vi "Test HTTPS.vi"() -> ()   [LabVIEW 2020]
uses:
  lv-http-server/HTTP Server/Trace Log.ctl
  lv-http-server/HTTP Server/Trace Item.ctl
  lv-http-server/HTTP Server/Processing Step.ctl
  lv-http-util/HTTP Utils/Method.ctl
  lv-http-server/HTTP Server/HTTPS Options.ctl
  Test HTTPS Controller/Test HTTPS Controller.lvclass
  C:/dev/lv20CE/relink/lv-http-server/HTTP Server/Handler/Handler.lvclass
  lv-http-server/HTTP Server/Server/Add Connection Handler.vi
  lv-http-server/HTTP Server/Server/Add Request Handler.vi
  lv-http-server/HTTP Server/Server/Add Route Handler.vi
  lv-http-server/HTTP Server/Server/Add Controller Handler.vi
  lv-http-server/HTTP Server/Server/Add Controller.vi
  lv-http-server/HTTP Server/Server/Add Response Handler.vi
  lv-http-server/HTTP Server/Server/Add Complete Handler.vi
  lv-http-server/HTTP Server/Server/Add Exception Handler.vi
  lv-http-server/HTTP Server/Connection Handler/Connection Handler.lvclass
  lv-http-server/HTTP Server/Request Handler/Request Handler.lvclass
  lv-http-server/HTTP Server/Route Handler/Route Handler.lvclass
  lv-http-server/HTTP Server/Controller Handler/Controller Handler.lvclass
  lv-http-server/HTTP Server/Controller/Controller.lvclass
  lv-http-server/HTTP Server/Response Handler/Response Handler.lvclass
  lv-http-server/HTTP Server/Complete Handler/Complete Handler.lvclass
  lv-http-server/HTTP Server/Exception Handler/Exception Handler.lvclass
  lv-http-server/HTTP Server/Server/Server.lvclass
  lv-http-server/HTTP Server/Handler/Handler.lvclass
  lv-http-server/HTTP Server/RequestTraceLog/RequestTraceLog.lvclass
  lv-http-server/HTTP Server/HTTP Server.lvlib
  lv-http-util/HTTP Utils/HTTP Utils.lvlib
panel:
  in  "Public Chain":path=path "C:/dev/lv20CE/relink/lv-http-server-examples/Examples/HTTPS/cert.pem"
  out "error out":errorcluster
  in  "Debug":bool=TRUE
  in  "Refresh Traces":bool
  out "Traces":T1[](array[typedef])=[{"Items"=[{"Duration"=0.00019280000014987309, "Step"=enum."Connection", "Class"="", "Info"="Start Request Parsing", "Status"=FALSE, "Code"=0, "Time"=3234.2736639}, {"Duration"=104.21120999999994, "Step"=enum."Connection", "Class"="", "Info"="Request Initialized", "Status"=TRUE, "Code"=66, "Time"=3338.4848739}, {"Duration"=0.0007422999997288571, "Step"=enum."Connection", "Class"="HTTP Utils.lvlib:Response.lvclass", "Info"="Completed", "Status"=TRUE, "Code"=66, "Time"=3338.4856161999996}], "Client"="tcp://DAB-2020SP1x86.ni.corp.natinst.com:52788", "Target"="", "Response Type"="", "Processing"=0.0007728000000497559, "Status"=200, "Method"=enum."GET", "Content Type"="", "Request Headers"=[], "Parsing"=3338.4848739, "Waiting"=-3234.2736639, "Identity"="", "Loaded"=FALSE, "Created"=FALSE, "Destroyed"=FALSE, "Response Headers"=[], "Created"=0.0, "Expires"=0.0, "Roles"=[], "Sending"=0.0}, {"Items"=[{"Duration"=0.006463199999870994, "Step"=enum."Connection", "Class"="", "Info"="Start Request Parsing", "Status"=FALSE, "Code"=0, "Time"=3459.3199179}, {"Duration"=0.008297200000015437, "Step"=enum."Connection", "Class"="", "Info"="Request Initialized", "Status"=TRUE, "Code"=66, "Time"=3459.3282151}, {"Duration"=0.0001554000000396627, "Step"=enum."Connection", "Class"="HTTP Utils.lvlib:Response.lvclass", "Info"="Completed", "Status"=TRUE, "Code"=66, "Time"=3459.3283705}], "Client"="tcp://DAB-2020SP1x86.ni.corp.natinst.com:52995", "Target"="", "Response Type"="", "Processing"=0.00019930000007661874, "Status"=200, "Method"=enum."GET", "Content Type"="", "Request Headers"=[], "Parsing"=3459.3282151, "Waiting"=-3459.3199179, "Identity"="", "Loaded"=FALSE, "Created"=FALSE, "Destroyed"=FALSE, "Response Headers"=[], "Created"=0.0, "Expires"=0.0, "Roles"=[], "Sending"=0.0}] {"Sending" format="%_6f"; "Expires" format="%<%X %x>T"; "Created" format="%<%X %x>T"; "Waiting" format="%_6f"; "Parsing" format="%_6f"; "Processing" format="%_6f"; "Items"."Time" format="%.6f"; "Items"."Duration" format="%.6f"}
  in  "Private Key":path=path "C:/dev/lv20CE/relink/lv-http-server-examples/Examples/HTTPS/key.pem"
  in  "HTTPS Port":u16=443
  in  "HTTP Port":u16=80
  in  "Always Secure?":bool=TRUE
  # "Request"
  # "Response"
  # "Session"
  # "Auth"
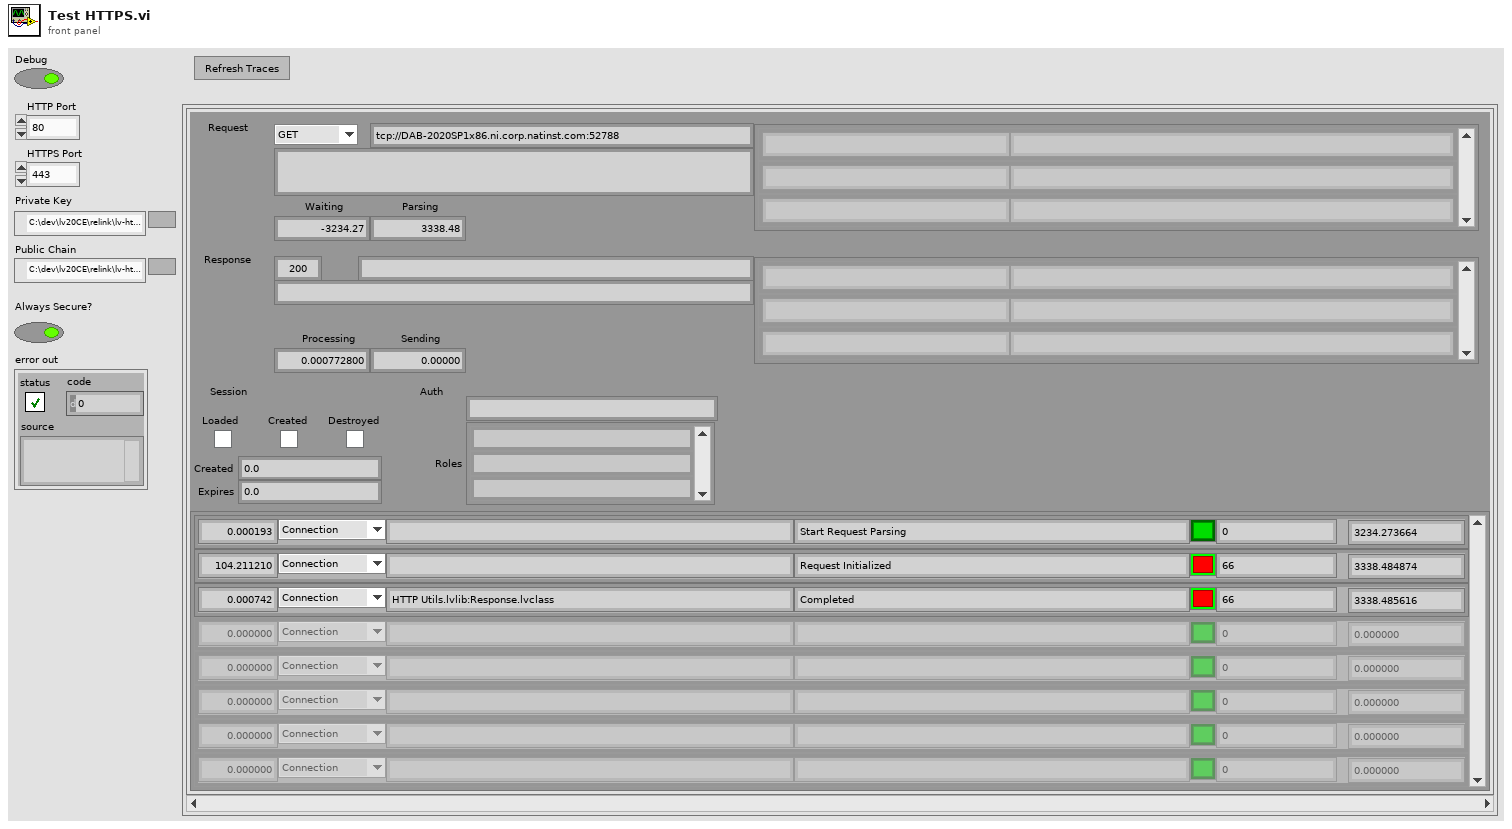
[diagram p1: front panel]
types:
  T1 = typedef "HTTP Server.lvlib/Trace Log.ctl" = cluster{"Items":T2[], "Client":string, "Target":string, "Response Type":string, "Processing":dbl, "Status":u16, "Method":T4, "Content Type":string, "Request Headers":cluster{"Name":string, "Value":string}[], "Parsing":dbl, "Waiting":dbl, "Identity":string, "Loaded":bool, "Created":bool, "Destroyed":bool, "Response Headers":cluster{"Name":string, "Value":string}[], "Created":dbl, "Expires":dbl, "Roles":string[], "Sending":dbl}
  T2 = typedef "HTTP Server.lvlib/Trace Item.ctl" = cluster{"Duration":dbl, "Step":T3, "Class":string, "Info":string, "Status":bool, "Code":i32, "Time":dbl}
  T3 = typedef "HTTP Server.lvlib/Processing Step.ctl" = enum16{"Connection", "Request", "Routing", "Controller Init", "Controller", "Response", "Complete", "Exception"}
  T4 = typedef "HTTP Utils.lvlib/Method.ctl" = enum16{"GET", "HEAD", "POST", "PUT", "DELETE", "CONNECT", "OPTIONS", "TRACE", "PATCH"}
  T5 = typedef "HTTP Server.lvlib/HTTPS Options.ctl" = cluster{"HTTPS Enabled":bool, "Private Key":path, "Private Key Format":enum32{"PKCS#8 (PEM)", "PKCS#8 (DER)"}, "Public Cert":path, "Public Cert Format":enum32{"X.509 (PEM)"}, "Always Secure?":bool, "HTTPS Port (443)":u16}
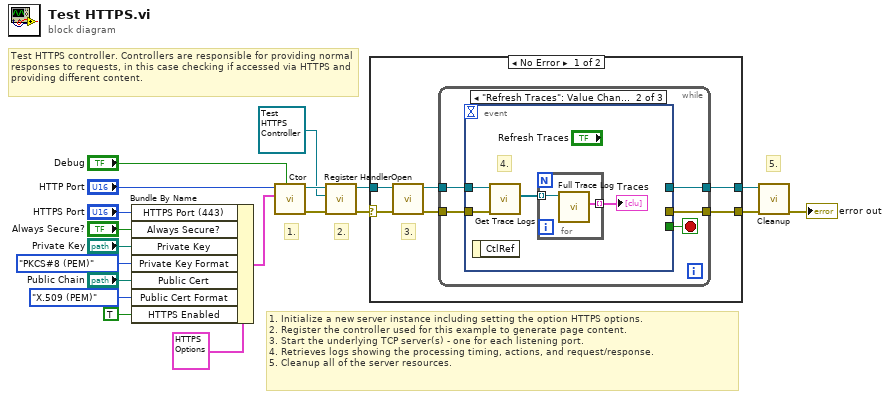
[diagram p0: block diagram]
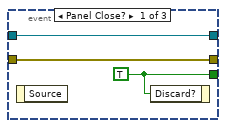
[diagram p2: hidden frame]
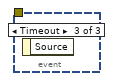
[diagram p3: hidden frame]
diagram:
  # "1. Initialize a new server instance including setting the option HTTPS options.\n2. Register the controller used for this example to generate page content.\n3. Start the underlying TCP server(s) - one for each listening port.\n4. Retrieves logs showing the processing timing, actions, and request/response.\n5. Cleanup all of the server resources."
  # "5."
  # "2."
  # "1."
  # "Test HTTPS controller. Controllers are responsible for providing normal responses to requests, in this case checking if accessed via HTTPS and providing different content."
  n1 = Bundle By Name(cluster=T5 {"HTTPS Enabled"=FALSE, "Private Key"=path "", "Private Key Format"=enum."PKCS#8 (PEM)", "Public Cert"=path "", "Public Cert Format"=enum."X.509 (PEM)", "Always Secure?"=TRUE, "HTTPS Port (443)"=433} ("HTTPS Options"), "HTTPS Port (443)"="HTTPS Port", "Always Secure?"="Always Secure?", "Private Key"="Private Key", "Private Key Format"=enum32{"PKCS#8 (PEM)", "PKCS#8 (DER)"}."PKCS#8 (PEM)", "Public Cert"="Public Chain", "Public Cert Format"=enum32{"X.509 (PEM)"}."X.509 (PEM)" ("Public Chain Format"), "HTTPS Enabled"=TRUE) -> (w4:T5)
  n2 = call "Ctor.vi"("Debug (F)"="Debug", "HTTPS Options (Disabled)"=w4, "HTTP Port (80)"="HTTP Port") -> ("error out"=w18:errorcluster, "Server out"=w19:refnum<class "Server.lvclass">)  [unwired: 7 in]
  n3 = call "Register Handler.vi"("error in (no error)"=w18, "Handler"=refnum<class "Test HTTPS Controller.lvclass"> refnum ("Test HTTPS Controller.lvclass"), "Server in"=w19) -> ("error out"=w1:errorcluster, "Server out"=w2:refnum<class "Server.lvclass">)  [unwired: 7 in]
  n4 = case shown="No Error" w1 {
    selector: w1 -> [w25 w41]
    tunnel: [w22 w40] -> w10
    tunnel: [w21 w41] -> w9
    tunnel: w2 -> [w20 w40]
    frame No Error {
      # "3."
      n5 = call "Open.vi"("error in (no error)"=w25, "Server in"=w20) -> ("error out"=w23:errorcluster, "Server out"=w24:refnum<class "Server.lvclass">)  [unwired: 8 in]
      n6 = while {
        tunnel: w24 -> [w28]
        tunnel: w23 -> [w29]
        tunnel: [w27] -> w22
        tunnel: [w26] -> w21
        stop <- w30 stop-if-true
        n7 = event shown="[1] \"Refresh Traces\": Value Change" {
          selector: _ -> [_ _ _]
          dyn-events: _ -> [_ _ _]
          timeout: _ -> [_ _ _]
          tunnel: [w31 _ _] -> w30
          tunnel: w29 -> [w32 w36 _]
          tunnel: w28 -> [w33 w37 _]
          tunnel: [w33 _ _] -> w27
          tunnel: [w32 _ _] -> w26
          event Panel Close? {
            w31 = TRUE ("Discard?")
            n8 = event-data() -> ()  [unwired: 1 in, 1 out]
            n9 = event-data("Discard?"=w31) -> ()  [unwired: 1 in, 1 out]
          }
          event "Refresh Traces": Value Change {
            # "4."
            n10 = event-data() -> ()  [unwired: 1 in, 1 out]
            n11 = call "Get Trace Logs.vi"("error in (no error)"=w36, "Server in"=w37) -> ("Trace Logs"=w35:refnum<class "RequestTraceLog.lvclass">[])  [unwired: 7 in, 2 out]
            n12 = for {
              tunnel: w35 -> [w39] mode=indexing
              tunnel: [w38] -> w34 mode=indexing
              n13 = call "Full Trace Log.vi"("RequestTraceLog in"=w39) -> ("Trace Log"=w38:T1)  [unwired: 8 in, 2 out]
            }
            "Traces" <- w34
          }
          event Timeout {
            n14 = event-data() -> ()  [unwired: 1 in, 1 out]
          }
        }
      }
    }
    frame Error {
    }
  }
  n15 = call "Cleanup.vi"("error in (no error)"=w9, "Server in"=w10) -> ("error out"=→"error out":errorcluster)  [unwired: 9 in]
